vi "window data for FFT start.vi"(7 "data in":dbl[](array[numeric]), 11 "Windowing ON":bool, 13 "Window type":enum16{"Hanning", "Hamming", "Blackman"}(ring)) -> (8 "windowed data out":dbl[](array[numeric]))   [LabVIEW 2019]
doc: "this subvi windows data so that the discontinuities at the edges of the data dont create an artificial response in the power spectrum"
uses:
  <vilib>/Analysis/4window.llb/Hanning Window (DBL).vi
  <vilib>/Analysis/4window.llb/Hamming Window (DBL).vi
  <vilib>/Analysis/4window.llb/Blackman Window (DBL).vi
  <vilib>/Analysis/4window.llb/AllCosWindow (DBL).vi
  <vilib>/Analysis/NI_AALPro.lvlib
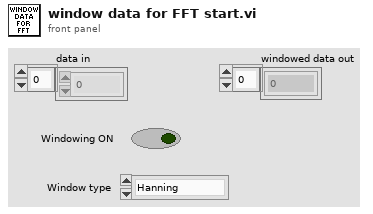
[diagram p1: front panel]
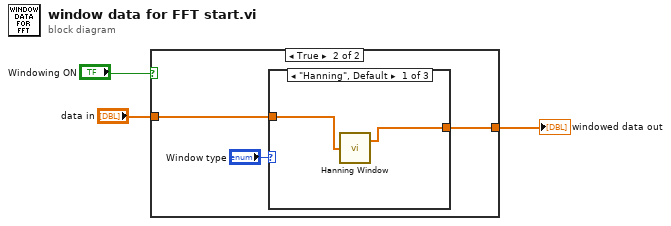
[diagram p0: block diagram]
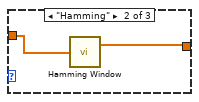
[diagram p3: hidden frame]
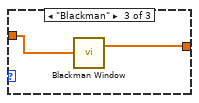
[diagram p4: hidden frame]
diagram:
  n1 = case shown="True" "Windowing ON" {
    tunnel: "data in" -> [w4 w6]
    tunnel: [w4 w5] -> w1
    frame False {
    }
    frame True {
      n2 = case shown="\"Hanning\", Default" "Window type" {
        tunnel: w6 -> [w9 w11 w13]
        tunnel: [w8 w10 w12] -> w5
        frame "Hanning", Default {
          n3 = call-poly <vilib>:"Hanning Window.vi"("X"=w9) -> ("Windowed X"=w8:dbl[])  [unwired: 1 out]
        }
        frame "Hamming" {
          n4 = call-poly <vilib>:"Hamming Window.vi"("X"=w11) -> ("Windowed X"=w10:dbl[])  [unwired: 1 out]
        }
        frame "Blackman" {
          n5 = call-poly <vilib>:"Blackman Window.vi"("X"=w13) -> ("Windowed X"=w12:dbl[])  [unwired: 1 out]
        }
      }
    }
  }
  "windowed data out" <- w1
